vi "daqOpcUaWriter.vi"(10 "DAQ Data Stream":dbl[](array[numeric]), 11 "OPC UA client refnum in":T1) -> ()   [LabVIEW 2017]
uses:
  <vilib>/OPCUA/controls/OPC UA Client Refnum.ctl
  <vilib>/OPCUA/controls/NodeIds.ctl
  <vilib>/OPCUA/controls/NodeId.ctl
  <vilib>/OPCUA/controls/Write Status.ctl
  <vilib>/OPCUA/client/Multiple Write Double.vi
  <vilib>/OPCUA/NI OPC UA Client.lvlib
panel:
  in  "Node Status":u16
  in  "Time Stamp":timestamp
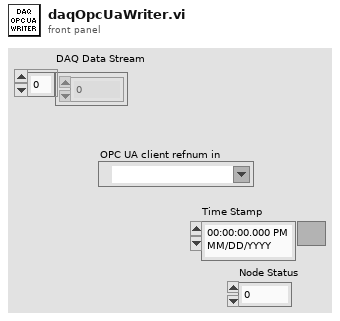
[diagram p1: front panel]
types:
  T1 = typedef "OPC UA Client Refnum.ctl" = refnum<k21>
  T2 = typedef "NodeIds.ctl" = T3[]
  T3 = typedef "NodeId.ctl" = string
  T4 = typedef "Write Status.ctl" = u32
  T5 = cluster{"node ID":T3, "value":dbl, "timestamp (current time)":timestamp, "node status":T4}
  T6 = cluster{"node ID":T3, "value":dbl, "timestamp (current time)":timestamp, "node status":T4}[]
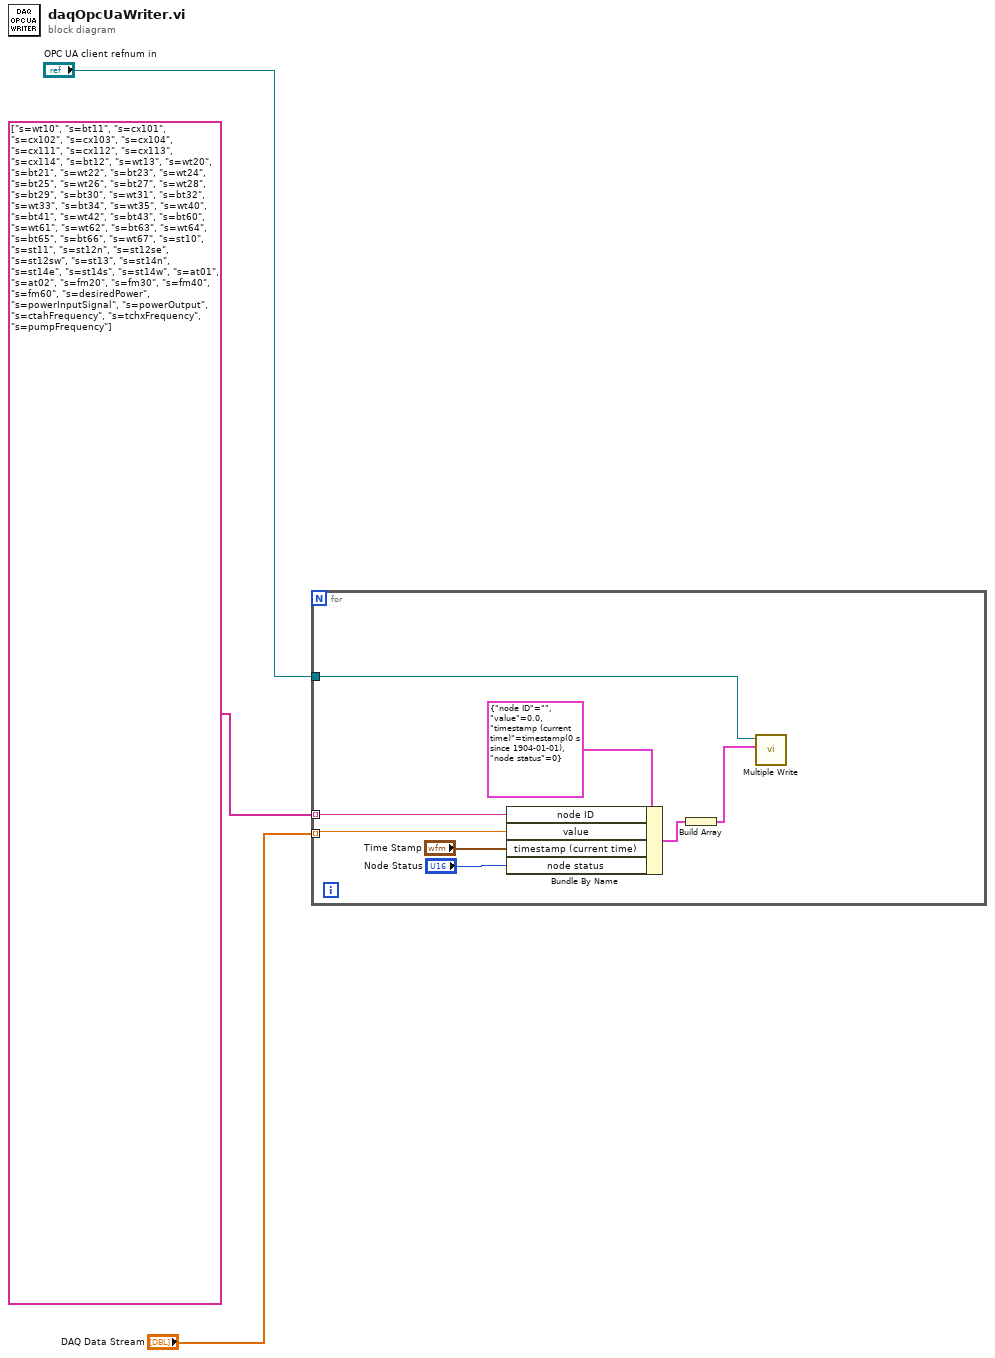
[diagram p0: block diagram]
diagram:
  n1 = for {
    tunnel: T2 ["s=wt10", "s=bt11", "s=cx101", "s=cx102", "s=cx103", "s=cx104", "s=cx111", "s=cx112", "s=cx113", "s=cx114", "s=bt12", "s=wt13", "s=wt20", "s=bt21", "s=wt22", "s=bt23", "s=wt24", "s=bt25", "s=wt26", "s=bt27", "s=wt28", "s=bt29", "s=bt30", "s=wt31", "s=bt32", "s=wt33", "s=bt34", "s=wt35", "s=wt40", "s=bt41", "s=wt42", "s=bt43", "s=bt60", "s=wt61", "s=wt62", "s=bt63", "s=wt64", "s=bt65", "s=bt66", "s=wt67", "s=st10", "s=st11", "s=st12n", "s=st12se", "s=st12sw", "s=st13", "s=st14n", "s=st14e", "s=st14s", "s=st14w", "s=at01", "s=at02", "s=fm20", "s=fm30", "s=fm40", "s=fm60", "s=desiredPower", "s=powerInputSignal", "s=powerOutput", "s=ctahFrequency", "s=tchxFrequency", "s=pumpFrequency"] ("node IDs") -> [w8] mode=indexing
    tunnel: "OPC UA client refnum in" -> [w7]
    tunnel: "DAQ Data Stream" -> [w6] mode=indexing
    n2 = Bundle By Name(cluster=T5 {"node ID"="", "value"=0.0, "timestamp (current time)"=timestamp(0 s since 1904-01-01), "node status"=0} ("request"), "node ID"=w8, "value"=w6, "timestamp (current time)"="Time Stamp", "node status"="Node Status") -> (w9:T5)
    n3 = Build Array(w9) -> (w4:T6)
    n4 = call-poly <vilib>:"Multiple Write.vi"("requests"=w4, "OPC UA client refnum in"=w7) -> ()  [unwired: 6 in, 4 out]
  }
